vi "Image_Processing.vi"(0 "Image":T1, 1 "input cluster":T2={"Mode"=enum."ROI", "Manual LUT"={"Minimum"=0.0, "Maximum"=0.0}, "BCG Values"={"Brightness"=128.0, "Contrast"=45.0, "Gamma"=1.0}, "ImageProcessed"=refnum, "Image "=refnum, "Log?"=FALSE, "Auto?"=FALSE, "ROI"={"Global Rectangle"=[], "Contours"=[]}, "ROI Parameters"={"Count"=0.0, "Size(um)"=0.0}, "Image X"=0, "Image Y"=0, "Horizontal ROI"={"Global Rectangle"=[], "Contours"=[]}, "HROI Pos"=0, "Custom ROI"={"Global Rectangle"=[], "Contours"=[]}, "Intensity Graph"=[]} {"ROI Parameters"."Size(um)" min=0 max=255 step=0.1 format="%.2f"; "ROI Parameters"."Count" min=0 max=255 step=0.1 format="%.2f"}, 3 "WaveformGraph in":refnum<vi>, 5 "error in (no error)":errorcluster) -> (15 "output cluster":T2={"Mode"=enum."ROI", "Manual LUT"={"Minimum"=0.0, "Maximum"=0.0}, "BCG Values"={"Brightness"=128.0, "Contrast"=45.0, "Gamma"=1.0}, "ImageProcessed"=refnum, "Image "=refnum, "Log?"=FALSE, "Auto?"=FALSE, "ROI"={"Global Rectangle"=[], "Contours"=[]}, "ROI Parameters"={"Count"=0.0, "Size(um)"=0.0}, "Image X"=0, "Image Y"=0, "Horizontal ROI"={"Global Rectangle"=[], "Contours"=[]}, "HROI Pos"=0, "Custom ROI"={"Global Rectangle"=[], "Contours"=[]}, "Intensity Graph"=[]} {"ROI Parameters"."Size(um)" min=0 max=255 step=0.1 format="%.2f"; "ROI Parameters"."Count" min=0 max=255 step=0.1 format="%.2f"}, 16 "ROI Parameters":cluster{"Count":i32, "Size (um)":i32}, 17 "Image Processed":T1, 19 "error out":errorcluster)   [LabVIEW 2023, in "Camera_Controller.lvlib"]
uses:
  Camera_Controller.lvlib
  <vilib>/vision/Image Controls.llb/IMAQ Image.ctl
  typedefs/ImageProcessingParameters.ctl
  <vilib>/vision/NI_Vision_Development_Module.lvlib
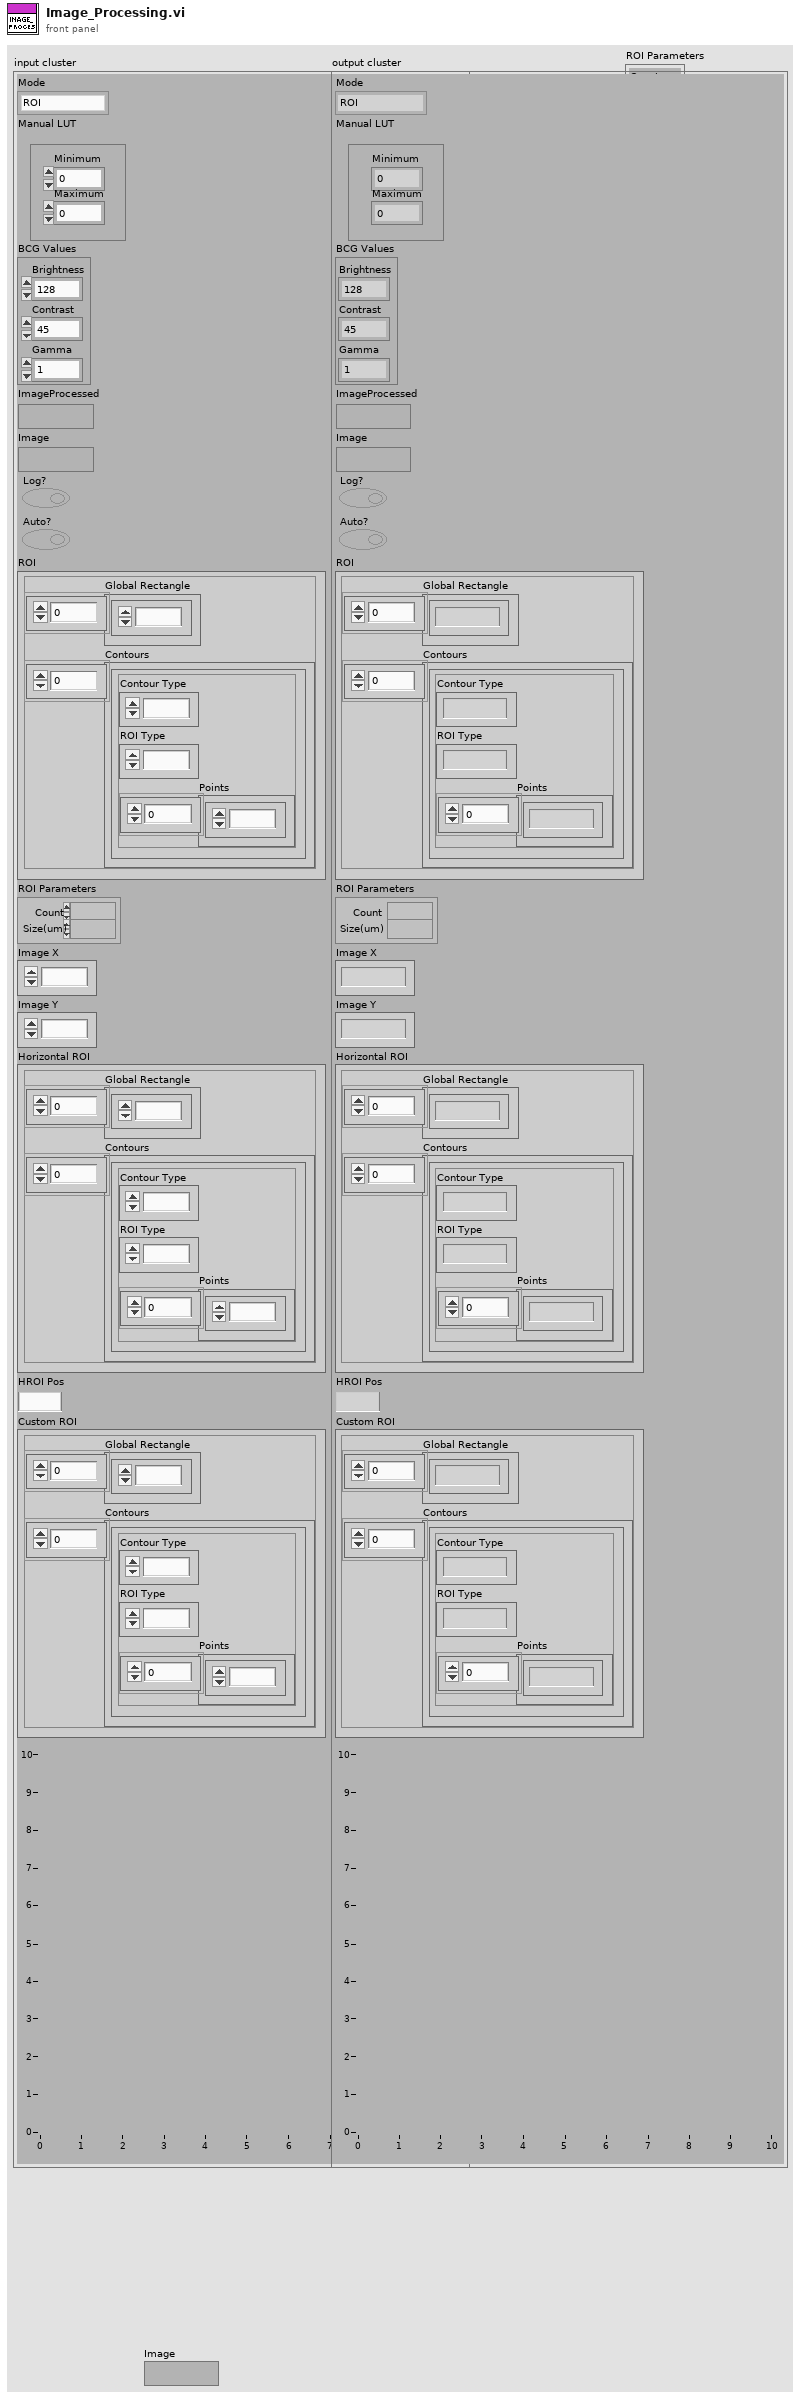
[diagram p1: front panel]
types:
  T1 = typedef "IMAQ Image.ctl" = refnum<image>
  T2 = typedef "ImageProcessingParameters.ctl" = cluster{"Mode":enum16{"ROI", "Image"}, "Manual LUT":cluster{"Minimum":dbl, "Maximum":dbl}, "BCG Values":cluster{"Brightness":sgl, "Contrast":sgl, "Gamma":sgl}, "ImageProcessed":T1, "Image ":T1, "Log?":bool, "Auto?":bool, "ROI":cluster{"Global Rectangle":i32[], "Contours":cluster{"Contour Type":u32, "ROI Type":u32, "Points":i32[]}[]}, "ROI Parameters":cluster{"Count":sgl, "Size(um)":sgl}, "Image X":i32, "Image Y":i32, "Horizontal ROI":cluster{"Global Rectangle":i32[], "Contours":cluster{"Contour Type":u32, "ROI Type":u32, "Points":i32[]}[]}, "HROI Pos":u16, "Custom ROI":cluster{"Global Rectangle":i32[], "Contours":cluster{"Contour Type":u32, "ROI Type":u32, "Points":i32[]}[]}, "Intensity Graph":u8[][]}
  T3 = cluster{"Brightness":sgl, "Contrast":sgl, "Gamma":sgl}
  T4 = cluster{"Global Rectangle":i32[], "Contours":cluster{"Contour Type":u32, "ROI Type":u32, "Points":i32[]}[]}
  T5 = cluster{"Lower value":sgl, "Upper value":sgl, "Replace Value":sgl, "Keep/Replace Value (Replace)":bool}[]
  T6 = enum32{"Linear", "Log", "Exp", "Square", "Square root", "Power X", "Power 1/X"}
  T7 = cluster{"Min":sgl, "Max":sgl, "Mean":sgl, "Std Dev":sgl, "Count":i32, "Size (um)":i32}
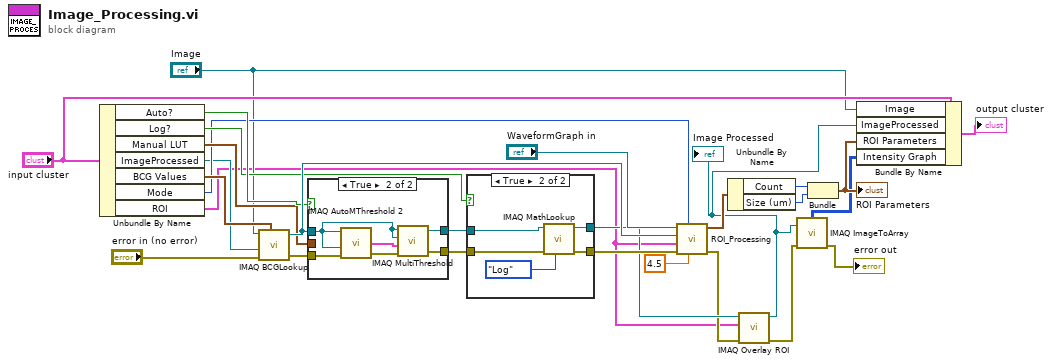
[diagram p0: block diagram]
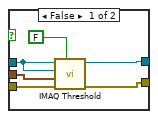
[diagram p3: hidden frame]
diagram:
  n1 = Unbundle By Name("input cluster") -> ("Auto?"=w18:bool, "Log?"=w15:bool, "Manual LUT"=w17:cluster{"Minimum":dbl, "Maximum":dbl}, "ImageProcessed"=w8:T1, "BCG Values"=w16:T3, "Mode"=w14:enum16{"ROI", "Image"}, "ROI"=w5:T4)
  n2 = call "IMAQ BCGLookup"("Image Src"="Image", "BCG Values"=w16, "Image Dst"=w8, "error in (no error)"="error in (no error)") -> ("Image Dst Out"=w25:T1, "error out"=w24:errorcluster)  [unwired: 3 in]
  n3 = case shown="True" w18 {
    tunnel: w25 -> [w30 w38]
    tunnel: [w32 w37] -> w22
    tunnel: w24 -> [w34 w40]
    tunnel: [w33 w35] -> w23
    tunnel: w17 -> [w31 _]
    frame False {
      n4 = call "IMAQ Threshold"("Keep/Replace Value (Replace)"=FALSE, "error in (no error)"=w34, "Range"=w31, "Image Dst"=w30, "Image Src"=w30) -> ("error out"=w33:errorcluster, "Image Dst Out"=w32:T1)  [unwired: 5 in]
    }
    frame True {
      n5 = call "IMAQ AutoMThreshold 2"("error in (no error)"=w40, "Image Mask"=w38, "Image"=w38) -> ("error out"=w36:errorcluster, "Threshold Data out"=w39:T5)  [unwired: 1 in, 1 out]
      n6 = call "IMAQ MultiThreshold"("error in (no error)"=w36, "Threshold Data"=w39, "Image Dst"=w38, "Image Src"=w38) -> ("error out"=w35:errorcluster, "Image Dst Out"=w37:T1)  [unwired: 1 in]
    }
  }
  n7 = case shown="True" w15 {
    tunnel: w22 -> [w41 w46]
    tunnel: w23 -> [w42 w45]
    tunnel: [w42 w44] -> w13
    tunnel: [w41 w43] -> w7
    frame False {
    }
    frame True {
      n8 = call "IMAQ MathLookup"("Operator"=T6."Log", "error in (no error)"=w45, "Image Src"=w46) -> ("error out"=w44:errorcluster, "Image Dst Out"=w43:T1)  [unwired: 7 in]
    }
  }
  n9 = call "ROI_Processing.vi"("Pixel Size(um)"=4.5, "Histogram Mode"=w14, "error in (no error)"=w13, "ROI"=w5, "Image Dst Out"=w25, "WaveformGraph in"="WaveformGraph in") -> ("error out"=w6:errorcluster, "ROI Pixel Statistics"=w19:T7)  [unwired: 4 in]
  n10 = Unbundle By Name(w19) -> ("Count"=w20:i32, "Size (um)"=w21:i32)
  n11 = call "IMAQ Overlay ROI"("error in (no error)"=w6, "ROI Descriptor"=w5, "Image"=w7) -> ("error out"=w2:errorcluster, "Image Out"=w3:T1)  [unwired: 7 in]
  "Image Processed" <- w3
  n12 = call "IMAQ ImageToArray"("error in (no error)"=w2, "Image"=w3) -> ("error out"=→"error out":errorcluster, "Image Pixels (U8)"=w4:u8[][])  [unwired: 2 in, 3 out]
  n13 = Bundle("Count"=w20, "Size (um)"=w21) -> (w11:cluster{"Count":i32, "Size (um)":i32})  [unwired: 1 in]
  "ROI Parameters" <- w11
  n14 = Bundle By Name(cluster="input cluster", "Image"="Image", "ImageProcessed"=w3, "ROI Parameters"=w11, "Intensity Graph"=w4) -> (→"output cluster":T2)
